vi "Kommunikation Alarme.vi"(8 "error in (no error)":errorcluster caption="Fehler (Eingang, kein Fehler)", 11 "Steuerung PNS Eingang":refnum<class "Steuerung PNS.lvclass">) -> (0 "error out":errorcluster caption="Fehler (Ausgang)", 2 "Werte":cluster{u16[], u16[]}, 3 "Steuerung PNS Ausgang":refnum<class "Steuerung PNS.lvclass">)   [LabVIEW 2020, in "Steuerung PNS.lvclass"]
doc: "Kommuniziert mit der Steuerung, um die Alarme auszulesen und speichert diese im Objekt.\nDie Istwerte werden mit den Sollwerten verglichen und bei Unterschieden die Werte zum schreiben (Adresse/Wert Cluster) werden auch im Objekt gespeichert und gelichzeitig als Output zur Verfügung gestellt.\n(automatisch je nach Steuerungstype werden die richtigen Adressen verwendet - durch die transparente SubKlasse)\n(Implementierung des Ist Soll Vergleichs in der jeweiligen SubKlasse)\nRIW"
uses:
  Steuerung PNS.lvclass
  Steuerung PNS.lvclass/Steuerung PNS.ctl
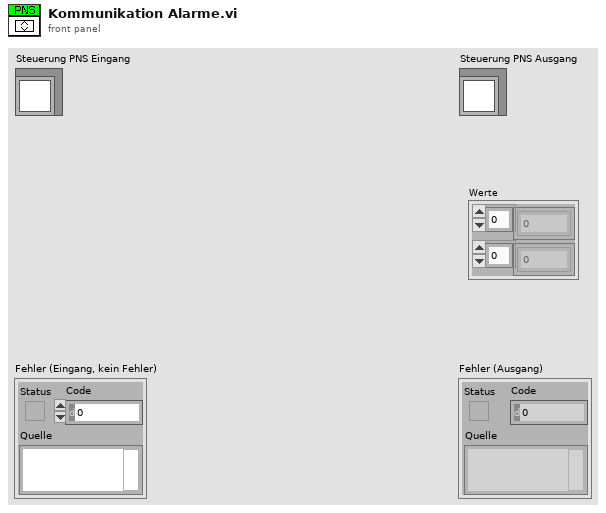
[diagram p1: front panel]
types:
  T1 = typedef "Steuerung PNS.lvclass/Adresse.ctl" = cluster{i32[][], i32}
  T2 = typedef "Steuerung PNS.lvclass/Werte.ctl" = cluster{"Adressen":u16[], "Werte":u16[]}
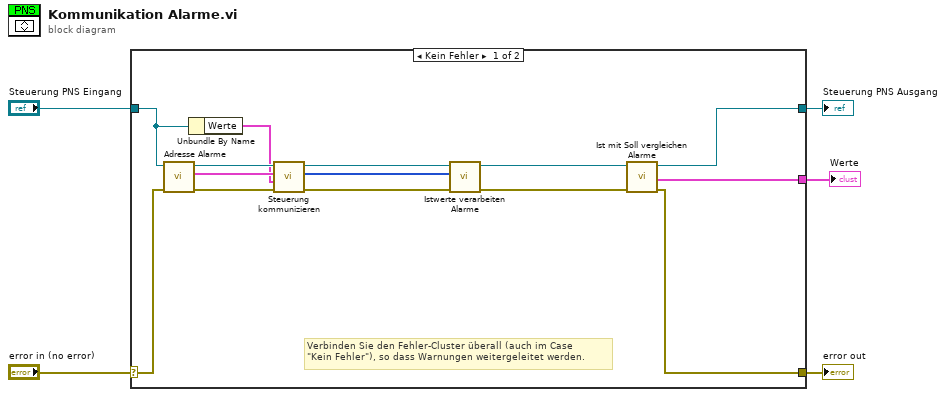
[diagram p0: block diagram]
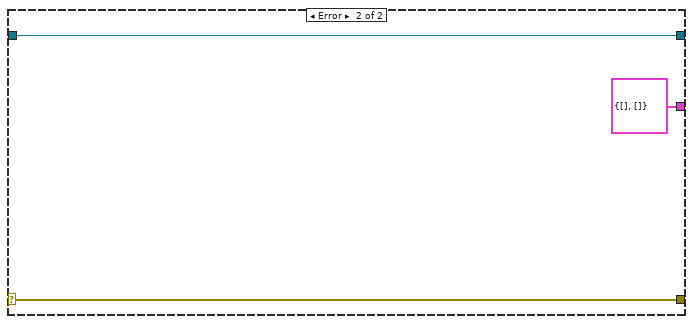
[diagram p2: hidden frame]
diagram:
  n1 = case shown="Kein Fehler" "error in (no error)" {
    selector: "error in (no error)" -> [w8 w22]
    tunnel: [w7 w22] -> w4
    tunnel: [w9 w21] -> w2
    tunnel: "Steuerung PNS Eingang" -> [w10 w21]
    tunnel: [w6 cluster{u16[], u16[]} {[], []} ("Werte")] -> w1
    frame No Error {
      # "Verbinden Sie den Fehler-Cluster überall (auch im Case\n\"Kein Fehler\"), so dass Warnungen weitergeleitet werden."
      n2 = call-dynamic "Adresse Alarme.vi"("error in (no error)"=w8, "Steuerung PNS Eingang"=w10) -> ("error out"=w17:errorcluster, "Adressen"=w18:T1, "Steuerung PNS Ausgang"=w19:refnum<class "Steuerung PNS.lvclass">)  [unwired: 7 in]
      n3 = Unbundle By Name(w10) -> ("Werte"=w16:T2)
      n4 = call "Steuerung kommunizieren.vi"("Steuerung PNS Eingang"=w19, "Adressen"=w18, "Werte"=w16, "error in (no error)"=w17) -> ("Steuerung PNS Ausgang"=w15:refnum<class "Steuerung PNS.lvclass">, "Istwerte"=w14:u16[], "error out"=w13:errorcluster)  [unwired: 4 in]
      n5 = call-dynamic "Istwerte verarbeiten Alarme.vi"("error in (no error)"=w13, "Istwerte"=w14, "Steuerung PNS Eingang"=w15) -> ("error out"=w11:errorcluster, "Steuerung PNS Ausgang"=w12:refnum<class "Steuerung PNS.lvclass">)  [unwired: 7 in]
      n6 = call-dynamic "Ist mit Soll vergleichen Alarme.vi"("error in (no error)"=w11, "Steuerung PNS Eingang"=w12) -> ("error out"=w7:errorcluster, "Werte"=w6:cluster{u16[], u16[]}, "Steuerung PNS Ausgang"=w9:refnum<class "Steuerung PNS.lvclass">)  [unwired: 7 in]
    }
    frame Error {
    }
  }
  "error out" <- w4
  "Steuerung PNS Ausgang" <- w2
  "Werte" <- w1
